vi "Create Directory.vi"(8 "error in (no error)":errorcluster, 10 "Remote Directory":string, 11 "FTP in":refnum<class "FTP.lvclass">) -> (0 "error out":errorcluster, 3 "FTP out":refnum<class "FTP.lvclass">)   [LabVIEW 2017, in "FTP.lvlib" / "FTP.lvclass"]
doc: "This vi will create a directory on the FTP server. The directory to be created is specified by the Remote Directory parameter."
uses:
  FTP.lvclass
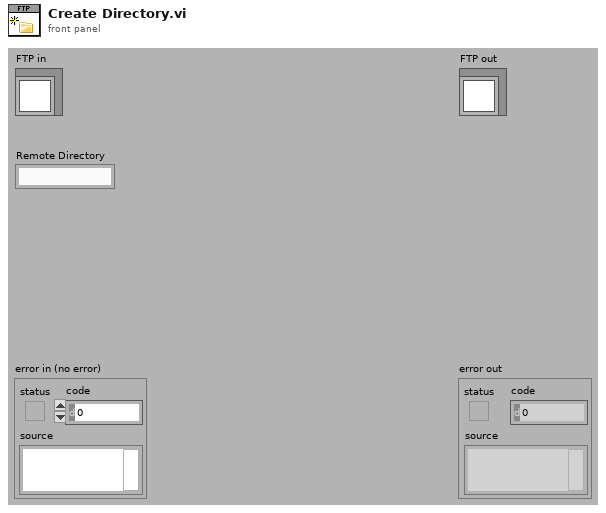
[diagram p1: front panel]
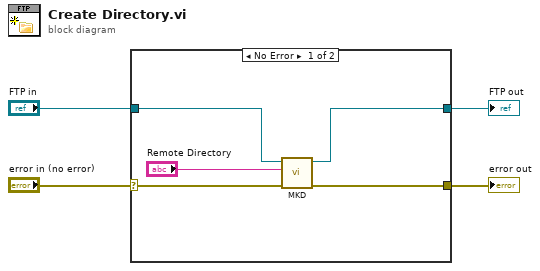
[diagram p0: block diagram]
diagram:
  n1 = case shown="No Error" "error in (no error)" {
    selector: "error in (no error)" -> [w8 w11]
    tunnel: [w6 w11] -> w3
    tunnel: [w7 w10] -> w1
    tunnel: "FTP in" -> [w9 w10]
    frame No Error {
      n2 = call "MKD.vi"("error in (no error)"=w8, "Remote Directory"="Remote Directory", "FTP in"=w9) -> ("error out"=w6:errorcluster, "FTP out"=w7:refnum<class "FTP.lvclass">)  [unwired: 7 in]
    }
    frame Error {
    }
  }
  "error out" <- w3
  "FTP out" <- w1
